vi "integral_ctrl.vi"(6 "Mode":T1=enum."Tustin (Bilinear)", 7 "Initialize?":bool, 8 "Sampling \nTime":dbl, 9 "Anti-windup limits":cluster{"Lower limit":dbl, "Upper limit":dbl}={"Lower limit"=-10.0, "Upper limit"=10.0}, 10 "Ki":dbl=1.0, 11 "Input":dbl) -> (0 "Sampling\nTime Out":dbl, 3 "Output":dbl)   [LabVIEW 2018, in "DiscreteControllers.lvlib"]
doc: "Integral controller implementation\nImplements: Ki/s in discrete time.\nSelect the discretization scheme appropriately.\nAnti-windup limits can be specified as needed."
uses:
  DiscreteControllers.lvlib
  TF_diff_mode.ctl
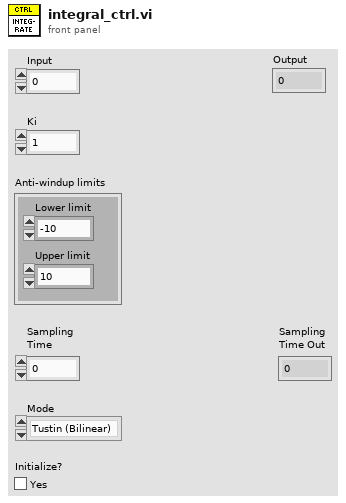
[diagram p1: front panel]
types:
  T1 = typedef "DiscreteControllers.lvlib/TF_diff_mode.ctl" = enum16{"Forward Euler", "Backward Euler", "Tustin (Bilinear)"}
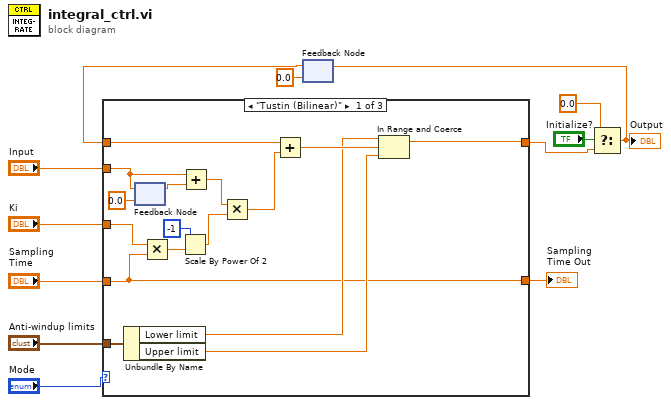
[diagram p0: block diagram]
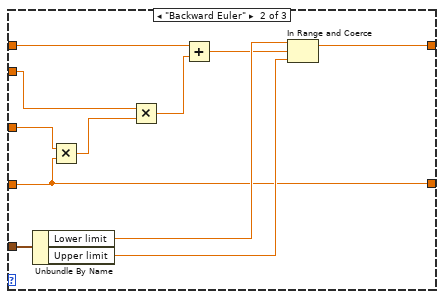
[diagram p2: hidden frame]
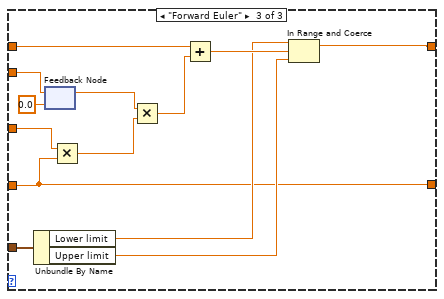
[diagram p3: hidden frame]
diagram:
  n1 = feedback #1(0.0 ("Output")) -> (w10:dbl)
  n2 = case shown="\"Tustin (Bilinear)\"" "Mode" {
    tunnel: w10 -> [w20 w32 w47]
    tunnel: "Input" -> [w27 w31 w45]
    tunnel: "Ki" -> [w25 w34 w43]
    tunnel: "Sampling \nTime" -> [w13 w33 w42]
    tunnel: [w14 w35 w46] -> w3
    tunnel: "Anti-windup limits" -> [w17 w29 w40]
    tunnel: [w13 w33 w42] -> w6
    frame "Tustin (Bilinear)" {
      n3 = Unbundle By Name(w17) -> ("Lower limit"=w16:dbl, "Upper limit"=w15:dbl)
      n4 = feedback-in #2(w27) -> ()
      n5 = feedback #2(0.0 ("Input")) -> (w26:dbl)
      n6 = Multiply(x=w25, y=w13) -> (x*y=w24:dbl)
      n7 = Scale By Power Of 2(n=i16 -1, x=w24) -> (x*2^n=w21:dbl)
      n8 = Add(x=w27, y=w26) -> (x+y=w22:dbl)
      n9 = Multiply(x=w22, y=w21) -> (x*y=w19:dbl)
      n10 = Add(x=w20, y=w19) -> (x+y=w18:dbl)
      n11 = In Range and Coerce(upper limit=w16, x=w18, lower limit=w15) -> (coerced(x)=w14:dbl)  [unwired: 1 out]
    }
    frame "Backward Euler" {
      n12 = Unbundle By Name(w29) -> ("Lower limit"=w38:dbl, "Upper limit"=w39:dbl)
      n13 = Multiply(x=w34, y=w33) -> (x*y=w30:dbl)
      n14 = Multiply(x=w31, y=w30) -> (x*y=w36:dbl)
      n15 = Add(x=w32, y=w36) -> (x+y=w37:dbl)
      n16 = In Range and Coerce(upper limit=w38, x=w37, lower limit=w39) -> (coerced(x)=w35:dbl)  [unwired: 1 out]
    }
    frame "Forward Euler" {
      n17 = Unbundle By Name(w40) -> ("Lower limit"=w49:dbl, "Upper limit"=w48:dbl)
      n18 = feedback #3(0.0 ("Input")) -> (w44:dbl)
      n19 = feedback-in #3(w45) -> ()
      n20 = Multiply(x=w43, y=w42) -> (x*y=w41:dbl)
      n21 = Multiply(x=w44, y=w41) -> (x*y=w51:dbl)
      n22 = Add(x=w47, y=w51) -> (x+y=w50:dbl)
      n23 = In Range and Coerce(upper limit=w49, x=w50, lower limit=w48) -> (coerced(x)=w46:dbl)  [unwired: 1 out]
    }
  }
  "Sampling\nTime Out" <- w6
  n24 = Select(t=0.0, s="Initialize?", f=w3) -> (s? t:f=w2:dbl)
  "Output" <- w2
  n25 = feedback-in #1(w2) -> ()
